vi "运维调试_CODCr.vi"() -> ()   [LabVIEW 2016, in "CodCr.lvlib"]
uses:
  CodCr.lvlib
  <vilib>/Utility/miscctls.llb/LVPointTypeDef.ctl
  <vilib>/Plasmionique/MB Master/MB_Master_Serial/MB_Master_Serial.lvclass
  F:/Program Files/National Instruments/LabVIEW 2016/vi.lib/Plasmionique/MB Master/MB_Master/MB_Master.lvclass
  <vilib>/Plasmionique/MB Master/MB Master.lvlib
panel:
  out "文本.文本":string
  out "status":bool
  out "启动测量模式":T1(ring)
  out "曲线斜率B":sgl
  out "曲线斜率K":sgl
  out "量程上限":sgl
  out "量程下限":sgl
  out "消解时长":u16
  out "消解温度":u16
  out "测量精度":u16
  out "测量结果":sgl
  out "标样参考值":sgl
  out "量程":u16
  out "工作状态":T1(ring)
  out "仪器时间":timestamp
  out "关键参数区":T2
  out "状态告警区":T3
  out "测量数据区":T4 {"单位" items=["ug/L", "mg/L", "ppm", "mg/m3", "cm", "ppb", "ug/m3", "%", "nmol/mol", "umol/mol", "MPN/L", "MPN/100ml", "ng/m3", "NTU", "无量纲", "ms/cm", "us/cm", "℃", "mV", "万个/L"]}
  out "error out":errorcluster
  out "系统时间":timestamp
  in  "VISA Resource":refnum<visa-resource-name>="COM8"
  out "Registers":u16[](array[numeric])
  in  "枚举":enum16{"读取", "写入", "读取参数"}(ring)
  in  "停止":bool
  in  "校时":bool
  in  "标样校准":bool
  in  "空白校准":bool
  in  "零点核查":bool
  in  "标样核查":bool
  in  "水样测试":bool
  in  "返回":bool
  in  "设置":bool
  # "mg/L"
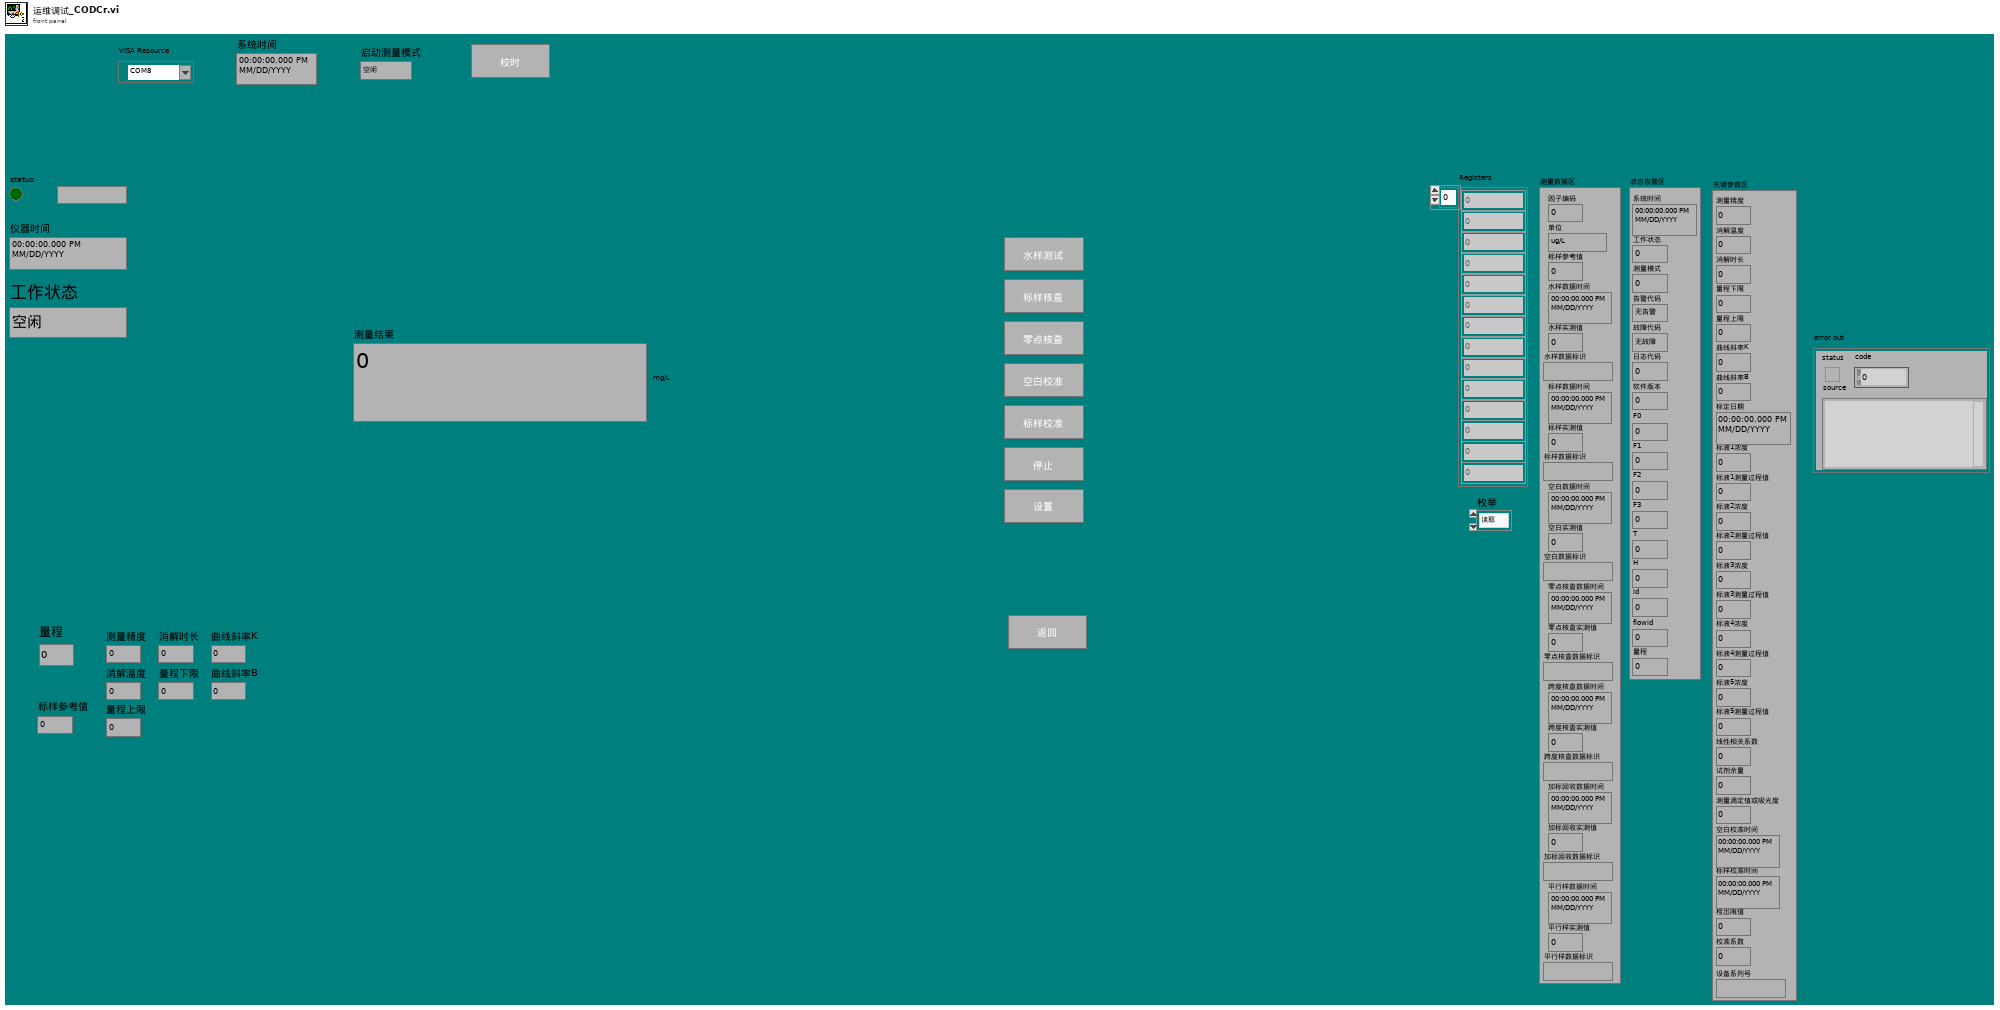
[diagram p1: front panel]
types:
  T1 = enum16{"空闲", "水样测试", "标样核查", "零点核查", "跨度核查", "空白测试", "平行样测试", "加标回收", "空白校准", "标样校准", "初始化（清洗）"}
  T2 = cluster{"测量精度":u16, "消解温度":u16, "消解时长":u16, "量程下限":sgl, "量程上限":sgl, "曲线斜率K":sgl, "曲线斜率B":sgl, "标定日期":timestamp, "标液1浓度":sgl, "标液1测量过程值":sgl, "标液2浓度":sgl, "标液2测量过程值":sgl, "标液3浓度":sgl, "标液3测量过程值":sgl, "标液4浓度":sgl, "标液4测量过程值":sgl, "标液5浓度":sgl, "标液5测量过程值":sgl, "线性相关系数":sgl, "试剂余量":u32, "测量滴定值或吸光度":sgl, "空白校准时间":timestamp, "标样校准时间":timestamp, "检出限值":sgl, "校准系数":sgl, "设备系列号":string}
  T3 = cluster{"系统时间":timestamp, "工作状态":u16, "测量模式":u16, "告警代码":enum16{"无告警", "缺试剂告警", "缺水样告警", "缺蒸馏水告警", "缺标液告警", "仪表漏液告警", "标定异常告警", "超量程告警", "加热异常", "低试剂预警", "超上限告警", "超下限告警", "仪表内部其他异常", "滴定异常告警", "电极异常告警", "量程切换告警", "参数设置告警", "PH电极电位异常", "电导率电极异常", "浊度光度异常", "溶解氧电极异常", "溶解氧光强异常", "温度异常告警", "PH异常告警", "溶解氧异常告警", "电导率异常告警", "浊度异常告警", "叶绿素异常告警", "藻密度异常告警", "蓝绿藻异常告警", "ORP异常告警", "氨氮异常告警", "清洁刷异常告警", "SD卡异常告警", "蓝牙异常告警", "Wifi异常告警", "流程异常告警"}, "故障代码":enum16{"无故障", "电机故障", "温度故障", "通讯故障", "滴定故障"}, "日志代码":u16, "软件版本":u16, "F0":sgl, "F1":sgl, "F2":sgl, "F3":sgl, "T":sgl, "H":sgl, "id":u16, "flowid":u16, "量程":u16}
  T4 = cluster{"因子编码":u32, "单位":u16, "标样参考值":sgl, "水样数据时间":timestamp, "水样实测值":sgl, "水样数据标识":string, "标样数据时间":timestamp, "标样实测值":sgl, "标样数据标识":string, "空白数据时间":timestamp, "空白实测值":sgl, "空白数据标识":string, "零点核查数据时间":timestamp, "零点核查实测值":sgl, "零点核查数据标识":string, "跨度核查数据时间":timestamp, "跨度核查实测值":sgl, "跨度核查数据标识":string, "加标回收数据时间":timestamp, "加标回收实测值":sgl, "加标回收数据标识":string, "平行样数据时间":timestamp, "平行样实测值":sgl, "平行样数据标识":string}
  T5 = cluster{"baud rate (bps)":u32, "stop bits":u16, "parity":u16, "flow control":u16, "timeout":u32, "retries":i32}
  T6 = cluster{"starting address":u16, "number of holding registers":u16}
  T7 = typedef "LVPointTypeDef.ctl" = cluster{"Horizontal":i16, "Vertical":i16}
  T8 = cluster{"时间标识":timestamp, "监测值":sgl, "单位":u16, "数据标识":string, "因子编码":u32, "标样参考值":sgl, "F0":sgl, "F1":sgl, "F2":sgl, "F3":sgl, "温度":sgl, "湿度":sgl, "量程标识":string}
  T9 = cluster{"系统时间":timestamp, "工作状态":enum16{"空闲", "水样测试", "标样核查", "零点核查", "跨度核查", "空白测试", "平行样测试", "加标回收", "空白校准", "标样校准", "初始化（清洗）"}, "测量模式":enum16{"待机", "连续模式", "周期模式", "定点模式", "受控模式", "手动模式"}, "告警代码":enum16{"无告警", "缺试剂告警", "缺水样告警", "缺蒸馏水告警", "缺标液告警", "仪表漏液告警", "标定异常告警", "超量程告警", "加热异常", "低试剂预警", "超上限告警", "超下限告警", "仪表内部其他异常", "滴定异常告警", "电极异常告警", "量程切换告警", "参数设置告警", "PH电极电位异常", "电导率电极异常", "浊度光度异常", "溶解氧电极异常", "溶解氧光强异常", "温度异常告警", "PH异常告警", "溶解氧异常告警", "电导率异常告警", "浊度异常告警", "叶绿素异常告警", "藻密度异常告警", "蓝绿藻异常告警", "ORP异常告警", "氨氮异常告警", "清洁刷异常告警", "SD卡异常告警", "蓝牙异常告警", "Wifi异常告警", "流程异常告警"}, "故障代码":enum16{"无故障", "电机故障", "温度故障", "通讯故障", "滴定故障"}, "日志代码":u16, "软件版本":u16, "F0":sgl, "F1":sgl, "F2":sgl, "F3":sgl, "T":sgl, "H":sgl, "id":u16, "flowid":u16, "量程":u16}
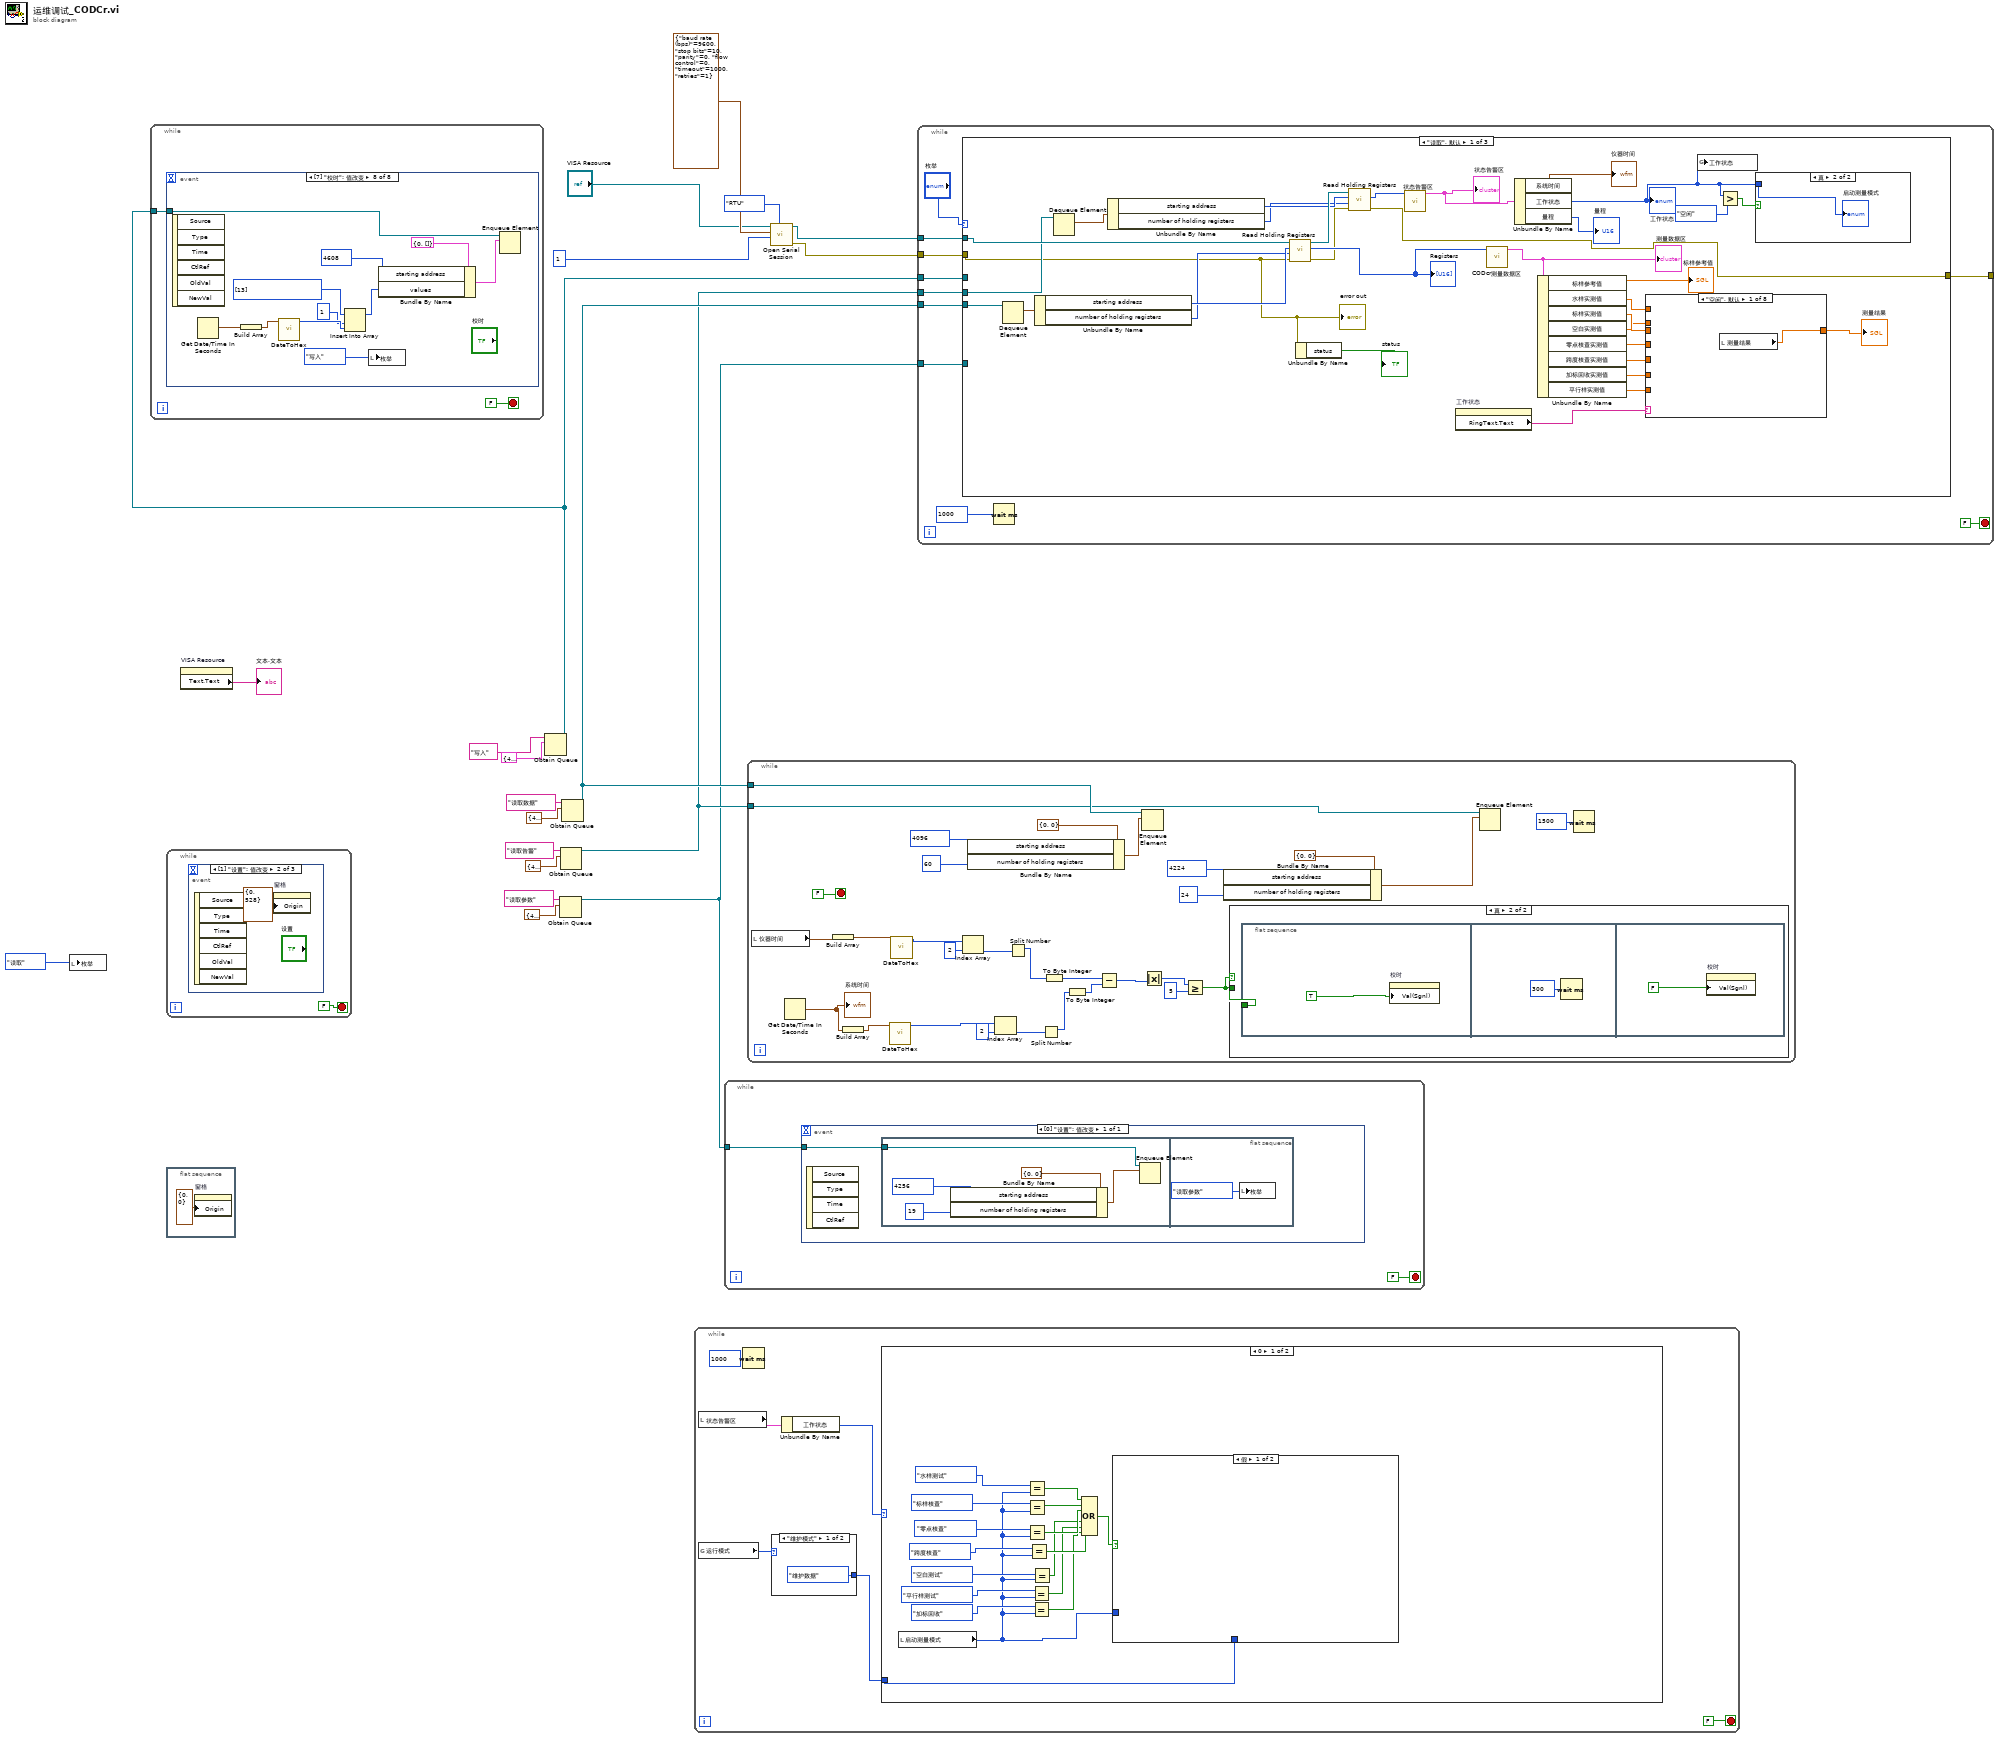
[diagram p0: block diagram]
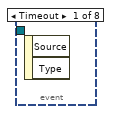
[diagram p3: hidden frame]
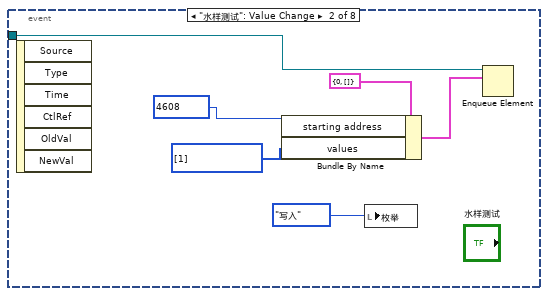
[diagram p4: hidden frame]
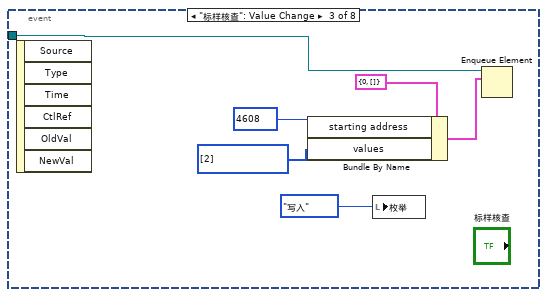
[diagram p5: hidden frame]
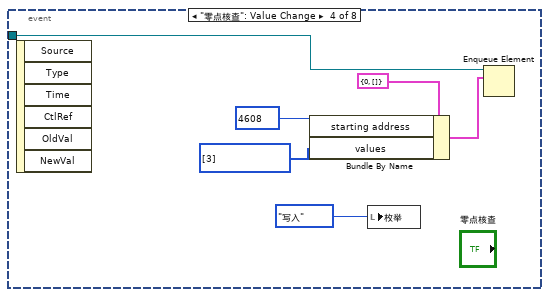
[diagram p6: hidden frame]
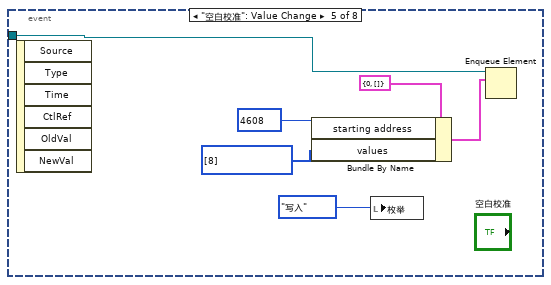
[diagram p7: hidden frame]
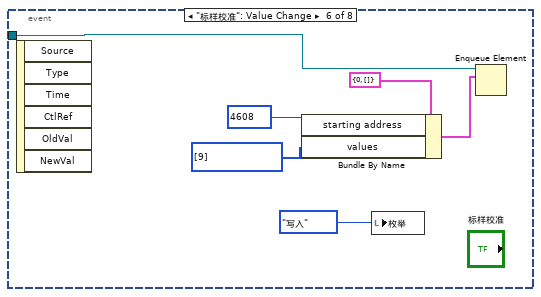
[diagram p8: hidden frame]
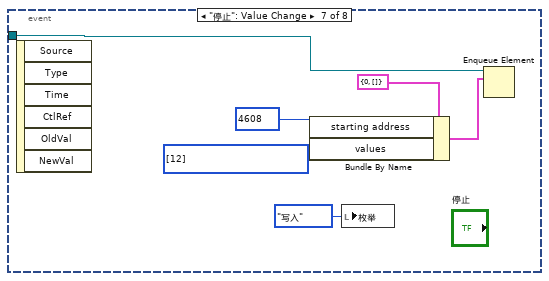
[diagram p9: hidden frame]
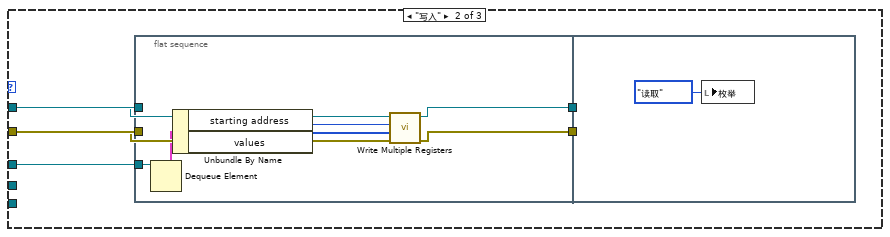
[diagram p18: hidden frame]
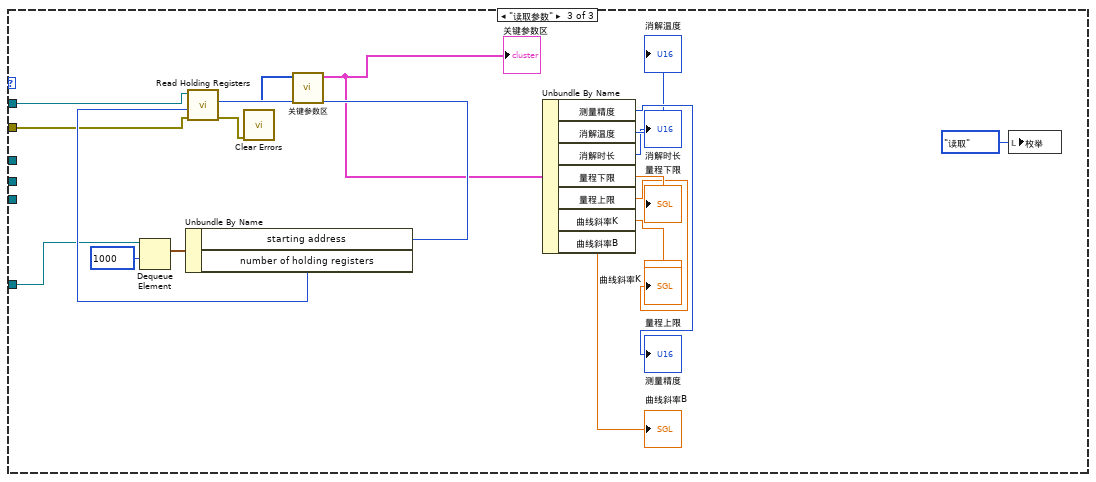
[diagram p19: hidden frame]
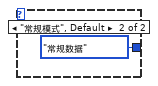
[diagram p20: hidden frame]
diagram:
  n1 = local write "枚举"(enum16{"读取", "写入"}."读取" ("枚举")) -> ()
  n2 = while {
    stop <- FALSE stop-if-true
    n3 = event shown="[1] \"设置\": 值改变" {
      selector: _ -> [_ _ _]
      dyn-events: _ -> [_ _ _]
      timeout: _ -> [_ _ _]
      event Timeout {
        n4 = event-data() -> ()  [unwired: 1 in, 3 out]
      }
      event "设置": Value Change {
        n5 = event-data() -> ()  [unwired: 1 in, 6 out]
        n6 = property on="窗格" class="Pane"("Origin"=T7 {"Horizontal"=0, "Vertical"=528} ("原点")) -> ()  [unwired: 2 in, 2 out]
      }
      event "返回": Value Change {
        n7 = event-data() -> ()  [unwired: 1 in, 6 out]
        n8 = property on="窗格" class="Pane"("Origin"=T7 {"Horizontal"=0, "Vertical"=0} ("原点")) -> ()  [unwired: 2 in, 2 out]
      }
    }
  }
  n9 = flat-sequence {
    frame #0 {
      n10 = property on="窗格" class="Pane"("Origin"=T7 {"Horizontal"=0, "Vertical"=0} ("原点")) -> ()  [unwired: 2 in, 2 out]
    }
  }
  n11 = property on="VISA Resource" class="VISAName"() -> ("Text.Text"=→"文本.文本":string)  [unwired: 2 in, 2 out]
  n12 = Obtain Queue(name (unnamed)="写入" ("名称（未命名）"), element data type=cluster{"starting address":u16, "values":u16[]} {"starting address"=4096, "values"=[]}) -> (queue out=w8:refnum<queue>)  [unwired: 3 in, 2 out]
  n13 = while {
    tunnel: w8 -> [w25]
    stop <- FALSE stop-if-true
    n14 = event shown="[7] \"校时\": 值改变" {
      selector: _ -> [_ _ _ _ _ _ _ _]
      dyn-events: _ -> [_ _ _ _ _ _ _ _]
      timeout: _ -> [_ _ _ _ _ _ _ _]
      tunnel: w25 -> [_ w32 w34 w40 w46 w52 w58 w70]
      event Timeout {
        n15 = event-data() -> ()  [unwired: 1 in, 2 out]
      }
      event "水样测试": Value Change {
        n16 = event-data() -> ()  [unwired: 1 in, 6 out]
        n17 = Bundle By Name(cluster=cluster{"starting address":u16, "values":u16[]} {"starting address"=0, "values"=[]} ("元素"), "starting address"=u16 4608, "values"=u16[] [1]) -> (w30:cluster{"starting address":u16, "values":u16[]})
        n18 = local write "枚举"(enum16{"读取", "写入"}."写入" ("枚举")) -> ()
        n19 = Enqueue Element(queue=w32, element=w30) -> ()  [unwired: 2 in, 3 out]
      }
      event "标样核查": Value Change {
        n20 = event-data() -> ()  [unwired: 1 in, 6 out]
        n21 = Bundle By Name(cluster=cluster{"starting address":u16, "values":u16[]} {"starting address"=0, "values"=[]} ("元素"), "starting address"=u16 4608, "values"=u16[] [2]) -> (w37:cluster{"starting address":u16, "values":u16[]})
        n22 = local write "枚举"(enum16{"读取", "写入"}."写入" ("枚举")) -> ()
        n23 = Enqueue Element(queue=w34, element=w37) -> ()  [unwired: 2 in, 3 out]
      }
      event "零点核查": Value Change {
        n24 = event-data() -> ()  [unwired: 1 in, 6 out]
        n25 = Bundle By Name(cluster=cluster{"starting address":u16, "values":u16[]} {"starting address"=0, "values"=[]} ("元素"), "starting address"=u16 4608, "values"=u16[] [3]) -> (w43:cluster{"starting address":u16, "values":u16[]})
        n26 = local write "枚举"(enum16{"读取", "写入"}."写入" ("枚举")) -> ()
        n27 = Enqueue Element(queue=w40, element=w43) -> ()  [unwired: 2 in, 3 out]
      }
      event "空白校准": Value Change {
        n28 = event-data() -> ()  [unwired: 1 in, 6 out]
        n29 = Bundle By Name(cluster=cluster{"starting address":u16, "values":u16[]} {"starting address"=0, "values"=[]} ("元素"), "starting address"=u16 4608, "values"=u16[] [8]) -> (w49:cluster{"starting address":u16, "values":u16[]})
        n30 = local write "枚举"(enum16{"读取", "写入"}."写入" ("枚举")) -> ()
        n31 = Enqueue Element(queue=w46, element=w49) -> ()  [unwired: 2 in, 3 out]
      }
      event "标样校准": Value Change {
        n32 = event-data() -> ()  [unwired: 1 in, 6 out]
        n33 = Bundle By Name(cluster=cluster{"starting address":u16, "values":u16[]} {"starting address"=0, "values"=[]} ("元素"), "starting address"=u16 4608, "values"=u16[] [9]) -> (w55:cluster{"starting address":u16, "values":u16[]})
        n34 = local write "枚举"(enum16{"读取", "写入"}."写入" ("枚举")) -> ()
        n35 = Enqueue Element(queue=w52, element=w55) -> ()  [unwired: 2 in, 3 out]
      }
      event "停止": Value Change {
        n36 = event-data() -> ()  [unwired: 1 in, 6 out]
        n37 = Bundle By Name(cluster=cluster{"starting address":u16, "values":u16[]} {"starting address"=0, "values"=[]} ("元素"), "starting address"=u16 4608, "values"=u16[] [12]) -> (w61:cluster{"starting address":u16, "values":u16[]})
        n38 = local write "枚举"(enum16{"读取", "写入", "读取参数"}."写入" ("枚举")) -> ()
        n39 = Enqueue Element(queue=w58, element=w61) -> ()  [unwired: 2 in, 3 out]
      }
      event "校时": Value Change {
        n40 = event-data() -> ()  [unwired: 1 in, 6 out]
        n41 = Get Date/Time In Seconds() -> (seconds since 1Jan1904=w68:timestamp)
        n42 = Build Array(w68) -> (w67:timestamp[])
        n43 = call "DateToHex.vi"("DATE"=w67) -> ("数组"=w65:u16[])  [unwired: 10 in]
        n44 = Insert Into Array(array=u16[] [13] ("values"), index=1 ("索引"), new element=w65) -> (w63:u16[])
        n45 = local write "枚举"(enum16{"读取", "写入"}."写入" ("枚举")) -> ()
        n46 = Bundle By Name(cluster=cluster{"starting address":u16, "values":u16[]} {"starting address"=0, "values"=[]} ("元素"), "starting address"=u16 4608, "values"=w63) -> (w72:cluster{"starting address":u16, "values":u16[]})
        n47 = Enqueue Element(queue=w70, element=w72) -> ()  [unwired: 2 in, 3 out]
      }
    }
  }
  n48 = Obtain Queue(name (unnamed)="读取参数" ("名称（未命名）"), element data type=T6 {"starting address"=4096, "number of holding registers"=100}) -> (queue out=w2:refnum<queue>)  [unwired: 3 in, 2 out]
  n49 = Obtain Queue(name (unnamed)="读取告警" ("名称（未命名）"), element data type=T6 {"starting address"=4096, "number of holding registers"=100}) -> (queue out=w5:refnum<queue>)  [unwired: 3 in, 2 out]
  n50 = Obtain Queue(name (unnamed)="读取数据" ("名称（未命名）"), element data type=T6 {"starting address"=4096, "number of holding registers"=100}) -> (queue out=w9:refnum<queue>)  [unwired: 3 in, 2 out]
  n51 = while {
    stop <- FALSE stop-if-true
    n52 = local read "状态告警区"() -> (w77:T3)
    n53 = global read "系统变量.vi" "运行模式"() -> (w75:enum16{"维护模式", "常规模式", "应急模式", "质控模式"})
    n54 = Wait (ms)(milliseconds to wait=u32 1000 ("等待时间（毫秒）")) -> ()  [unwired: 1 out]
    n55 = case shown="\"维护模式\"" w75 {
      tunnel: [enum16{"常规数据", "维护数据"}."维护数据" ("数据类型") enum16{"常规数据", "维护数据"}."常规数据" ("数据类型")] -> w74
      frame "维护模式" {
      }
      frame "常规模式", Default {
      }
    }
    n56 = Unbundle By Name(w77) -> ("工作状态"=w76:u16)
    n57 = case shown="0" w76 {
      tunnel: w74 -> [w98 _]
      frame 0 {
        n58 = local read "启动测量模式"() -> (w90:T1)
        n59 = Equal?(x=T1."水样测试" ("启动测量模式"), y=w90) -> (x = y?=w89:bool)
        n60 = Equal?(x=T1."标样核查" ("启动测量模式"), y=w90) -> (x = y?=w88:bool)
        n61 = Equal?(x=T1."零点核查" ("启动测量模式"), y=w90) -> (x = y?=w87:bool)
        n62 = Equal?(x=T1."跨度核查" ("启动测量模式"), y=w90) -> (x = y?=w86:bool)
        n63 = Equal?(x=T1."平行样测试" ("启动测量模式"), y=w90) -> (x = y?=w84:bool)
        n64 = Equal?(x=T1."加标回收" ("启动测量模式"), y=w90) -> (x = y?=w83:bool)
        n65 = Equal?(x=T1."空白测试" ("启动测量模式"), y=w90) -> (x = y?=w85:bool)
        n66 = Compound Arithmetic op=OR(w89, w88, w87, w86, w85, w84, w83) -> (w82:bool)
        n67 = case shown="假" w82 {
          tunnel: w90 -> [_ w104]
          tunnel: w98 -> [_ w103]
          frame False {
          }
          frame True {
            n68 = control-ref of="启动测量模式"() -> (w101:refnum<vi>)
            n69 = control-ref of="状态告警区"() -> (w99:refnum<vi>)
            n70 = control-ref of="测量数据区"() -> (w100:refnum<vi>)
            n71 = call "CODCr数据插入DATA (子VI).vi"("reference 2"=w99, "reference"=w100, "Enum输入"=w101) -> ("data"=w102:T8)  [unwired: 8 in]
            n72 = call "CODCr插入数据.vi"("database"="database1.mdb", "data"=w102, "table"="CODCr", "测量模式"=w104, "数据类型"=w103) -> ()  [unwired: 10 in, 1 out]
          }
        }
      }
      frame 1, Default {
      }
    }
  }
  n73 = while {
    tunnel: w2 -> [w107]
    stop <- FALSE stop-if-true
    n74 = event shown="[0] \"设置\": 值改变" {
      selector: _ -> [_]
      dyn-events: _ -> [_]
      timeout: _ -> [_]
      tunnel: w107 -> [w109]
      event "设置": Value Change {
        n75 = event-data() -> ()  [unwired: 1 in, 4 out]
        n76 = flat-sequence {
          tunnel: w109 -> [w110]
          frame #0 {
            n77 = Bundle By Name(cluster=T6 {"starting address"=0, "number of holding registers"=0} ("元素"), "starting address"=u16 4256, "number of holding registers"=u16 19) -> (w114:T6)
            n78 = Enqueue Element(queue=w110, element=w114) -> ()  [unwired: 2 in, 3 out]
          }
          frame #1 {
            n79 = local write "枚举"(enum16{"读取", "写入", "读取参数"}."读取参数" ("枚举")) -> ()
          }
        }
      }
    }
  }
  n80 = while {
    tunnel: w9 -> [w143]
    tunnel: w5 -> [w134]
    stop <- FALSE stop-if-true
    n81 = local read "仪器时间"() -> (w132:timestamp)
    n82 = Get Date/Time In Seconds() -> (seconds since 1Jan1904=w117:timestamp)
    "系统时间" <- w117
    n83 = Build Array(w132) -> (w133:timestamp[])
    n84 = Build Array(w117) -> (w116:timestamp[])
    n85 = call "DateToHex.vi"("DATE"=w116) -> ("数组"=w118:u16[])  [unwired: 10 in]
    n86 = call "DateToHex.vi"("DATE"=w133) -> ("数组"=w123:u16[])  [unwired: 10 in]
    n87 = Index Array(array=w123, index=2 ("索引")) -> (element=w121:u16)
    n88 = Bundle By Name(cluster=T6 {"starting address"=0, "number of holding registers"=0} ("元素"), "starting address"=u16 4096, "number of holding registers"=u16 60) -> (w141:T6)
    n89 = Index Array(array=w118, index=2 ("索引")) -> (element=w120:u16)
    n90 = Split Number(x=w121) -> (hi(x)=w127:u8)  [unwired: 1 out]
    n91 = Split Number(x=w120) -> (hi(x)=w124:u8)  [unwired: 1 out]
    n92 = To Byte Integer(number=w127) -> (8bit integer=w128:i8)
    n93 = To Byte Integer(number=w124) -> (8bit integer=w125:i8)
    n94 = Subtract(x=w128, y=w125) -> (x-y=w126:i8)
    n95 = Enqueue Element(queue=w143, element=w141) -> ()  [unwired: 2 in, 3 out]
    n96 = Absolute Value(x=w126) -> (abs(x)=w129:i8)
    n97 = Greater Or Equal?(x=w129, y=i8 5) -> (x >= y?=w131:bool)
    n98 = Bundle By Name(cluster=T6 {"starting address"=0, "number of holding registers"=0} ("元素"), "starting address"=u16 4224, "number of holding registers"=u16 24) -> (w135:T6)
    n99 = case shown="真" w131 {
      tunnel: w131 -> [_ w146]
      frame False {
      }
      frame True {
        n100 = flat-sequence {
          tunnel: w146 -> [_]
          frame #0 {
            n101 = property on="校时" class="Bool (严格)"("Val(Sgnl)"=TRUE ("时间校准")) -> ()  [unwired: 2 in, 2 out]
          }
          frame #1 {
            n102 = Wait (ms)(milliseconds to wait=u32 300 ("等待时间（毫秒）")) -> ()  [unwired: 1 out]
          }
          frame #2 {
            n103 = property on="校时" class="Bool (严格)"("Val(Sgnl)"=FALSE ("时间校准")) -> ()  [unwired: 2 in, 2 out]
          }
        }
      }
    }
    n104 = Enqueue Element(queue=w134, element=w135) -> ()  [unwired: 2 in, 3 out]
    n105 = Wait (ms)(milliseconds to wait=u32 1500 ("等待时间（毫秒）")) -> ()  [unwired: 1 out]
  }
  n106 = call <vilib>:"Open Serial Session.vi"("Mode (RTU)"=enum16{"RTU", "ASCII"}."RTU", "Slave ID"=u8 1, "Serial Config"=T5 {"baud rate (bps)"=9600, "stop bits"=10, "parity"=0, "flow control"=0, "timeout"=1000, "retries"=1}, "VISA Resource"="VISA Resource") -> ("Error out"=w18:errorcluster, "MB_Serial session"=w19:refnum<class "MB_Master_Serial.lvclass">)  [unwired: 6 in]
  n107 = while {
    tunnel: w19 -> [w157]
    tunnel: w18 -> [w156]
    tunnel: w8 -> [w155]
    tunnel: w9 -> [w154]
    tunnel: w5 -> [w153]
    tunnel: w2 -> [w151]
    tunnel: [w150] -> _
    stop <- FALSE stop-if-true
    n108 = case shown="\"读取\", 默认" "枚举" {
      tunnel: w157 -> [w192 w206 w225]
      tunnel: w156 -> [w163 w205 w224]
      tunnel: w155 -> [_ w204 _]
      tunnel: w154 -> [w191 _ _]
      tunnel: w153 -> [w186 _ _]
      tunnel: w151 -> [_ _ w226]
      tunnel: [w162 _ _] -> w150
      frame "读取", Default {
        n109 = Dequeue Element(queue=w191) -> (element=w190:T6)  [unwired: 2 in, 3 out]
        n110 = Unbundle By Name(w190) -> ("starting address"=w189:u16, "number of holding registers"=w188:u16)
        n111 = Dequeue Element(queue=w186) -> (element=w185:T6)  [unwired: 2 in, 3 out]
        n112 = Unbundle By Name(w185) -> ("starting address"=w182:u16, "number of holding registers"=w181:u16)
        n113 = call <vilib>:"Read Holding Registers.vi"("error in (no error)"=w163, "quantity"=w188, "starting address"=w189, "MB session in"=w192) -> ("error out"=w183:errorcluster, "Registers"=w187:u16[], "MB session out"=w184:refnum<class "MB_Master_Serial.lvclass">)  [unwired: 5 in]
        "Registers" <- w187
        n114 = Unbundle By Name(w163) -> ("status"=→"status":bool)
        n115 = call <vilib>:"Read Holding Registers.vi"("error in (no error)"=w183, "quantity"=w181, "starting address"=w182, "MB session in"=w184) -> ("error out"=w162:errorcluster, "Registers"=w180:u16[])  [unwired: 5 in, 1 out]
        n116 = call "状态告警区.vi"("数组"=w180) -> ("状态告警区"=w179:T9)  [unwired: 10 in]
        "状态告警区" <- w179
        n117 = property on="工作状态" class="Enum (严格)"() -> ("RingText.Text"=w172:string)  [unwired: 2 in, 2 out]
        n118 = call "CODcr测量数据区.vi"("数组"=w187) -> ("测量数据区"=w176:T4)  [unwired: 10 in]
        "测量数据区" <- w176
        n119 = Unbundle By Name(w179) -> ("系统时间"=→"仪器时间":timestamp, "工作状态"=w161:T1, "量程"=→"量程":u16)
        "工作状态" <- w161
        n120 = Unbundle By Name(w176) -> ("标样参考值"=→"标样参考值":sgl, "水样实测值"=w171:sgl, "标样实测值"=w169:sgl, "空白实测值"=w166:sgl, "零点核查实测值"=w168:sgl, "跨度核查实测值"=w167:sgl, "加标回收实测值"=w164:sgl, "平行样实测值"=w165:sgl)
        n121 = case shown="\"空闲\", 默认" w172 {
          tunnel: w171 -> [_ w194 _ _ _ _ _ _]
          tunnel: [w193 w194 w195 w196 w197 w198 w199 w200] -> w170
          tunnel: w169 -> [_ _ w195 _ _ _ _ _]
          tunnel: w168 -> [_ _ _ w196 _ _ _ _]
          tunnel: w167 -> [_ _ _ _ w197 _ _ _]
          tunnel: w166 -> [_ _ _ _ _ w198 _ _]
          tunnel: w165 -> [_ _ _ _ _ _ w199 _]
          tunnel: w164 -> [_ _ _ _ _ _ _ w200]
          frame "空闲", Default {
            n122 = local read "测量结果"() -> (w193:sgl)
          }
          frame "水样测试" {
          }
          frame "标样核查" {
          }
          frame "零点核查" {
          }
          frame "跨度核查" {
          }
          frame "空白测试" {
          }
          frame "平行样测试" {
          }
          frame "加标回收" {
          }
        }
        "测量结果" <- w170
        n123 = global write "CODCr工作状态.vi" "工作状态"(w161) -> ()
        n124 = Greater?(x=w161, y=T1."空闲") -> (0:w173:bool)
        n125 = case shown="真" w173 {
          tunnel: w161 -> [_ w201]
          frame False {
          }
          frame True {
            "启动测量模式" <- w201
          }
        }
        "error out" <- w163
      }
      frame "写入" {
        n126 = flat-sequence {
          tunnel: w206 -> [w214]
          tunnel: w205 -> [w213]
          tunnel: w204 -> [w210]
          tunnel: [w212] -> w203
          tunnel: [w211] -> w202
          tunnel: w203 -> [_]
          tunnel: w202 -> [_]
          frame #0 {
            n127 = Dequeue Element(queue=w210) -> (element=w209:cluster{"starting address":u16, "values":u16[]})  [unwired: 2 in, 3 out]
            n128 = Unbundle By Name(w209) -> ("starting address"=w208:u16, "values"=w207:u16[])
            n129 = call <vilib>:"Write Multiple Registers.vi"("error in (no error)"=w213, "values"=w207, "starting address"=w208, "MB session in"=w214) -> ("error out"=w211:errorcluster, "MB session out"=w212:refnum<class "MB_Master_Serial.lvclass">)  [unwired: 6 in]
          }
          frame #1 {
            n130 = local write "枚举"(enum16{"读取", "写入", "读取参数"}."读取" ("枚举")) -> ()
          }
        }
      }
      frame "读取参数" {
        n131 = Dequeue Element(queue=w226, timeout in ms (-1)=1000 ("超时毫秒(-1)")) -> (element=w233:T6)  [unwired: 1 in, 3 out]
        n132 = Unbundle By Name(w233) -> ("starting address"=w232:u16, "number of holding registers"=w231:u16)
        n133 = call <vilib>:"Read Holding Registers.vi"("error in (no error)"=w224, "quantity"=w231, "starting address"=w232, "MB session in"=w225) -> ("error out"=w228:errorcluster, "Registers"=w230:u16[])  [unwired: 5 in, 1 out]
        n134 = call <vilib>:"Clear Errors.vi"("error in (no error)"=w228) -> ()  [unwired: 5 in, 2 out]
        n135 = call "关键参数区.vi"("数组"=w230) -> ("关键参数区"=w227:T2)  [unwired: 10 in]
        "关键参数区" <- w227
        n136 = Unbundle By Name(w227) -> ("测量精度"=→"测量精度":u16, "消解温度"=→"消解温度":u16, "消解时长"=→"消解时长":u16, "量程下限"=→"量程下限":sgl, "量程上限"=→"量程上限":sgl, "曲线斜率K"=→"曲线斜率K":sgl, "曲线斜率B"=→"曲线斜率B":sgl)
        n137 = local write "枚举"(enum16{"读取", "写入", "读取参数"}."读取" ("枚举")) -> ()
      }
    }
    n138 = Wait (ms)(milliseconds to wait=u32 1000 ("等待时间（毫秒）")) -> ()  [unwired: 1 out]
  }
